vi "PH_ForceSensor.set GUI Refs.vi"(0 "VI in":refnum<vi>, 2 "GUI Refs":T1, 5 "error in (no error)":errorcluster) -> (14 "VI out":refnum<vi>, 19 "error out":errorcluster)   [LabVIEW 2014, in "PH_ForceSensor.lvlib"]
uses:
  PH_ForceSensor.lvlib
  PH_ForceSensor.GUI Refs.ctl
  PH_ForceSensor.Dataset.ctl
  PH_ForceSensor.Ranges.ctl
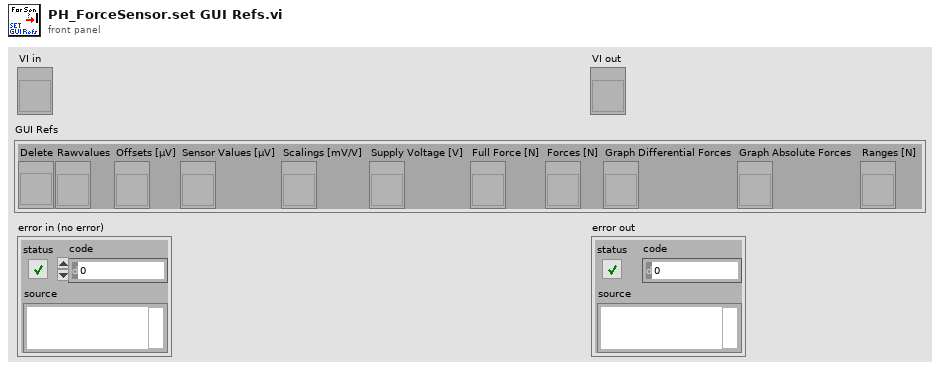
[diagram p1: front panel]
types:
  T1 = typedef "PH_ForceSensor.lvlib/PH_ForceSensor.GUI Refs.ctl" = cluster{"Delete":refnum<vi>, "Rawvalues":refnum<vi>, "Offsets [µV]":refnum<vi>, "Sensor Values [µV]":refnum<vi>, "Scalings [mV/V]":refnum<vi>, "Supply Voltage [V]":refnum<vi>, "Full Force [N]":refnum<vi>, "Forces [N]":refnum<vi>, "Graph Differential Forces":refnum<vi>, "Graph Absolute Forces":refnum<vi>, "Ranges [N]":refnum<vi>}
  T2 = typedef "PH_ForceSensor.lvlib/PH_ForceSensor.i attribute.ctl" = cluster{"GUI Refs":T1, "Rawvalues":T3, "Offsets [µV]":T3, "Scalings [mV/V]":T3, "Forces [N]":T3, "Supply Voltage [V]":dbl, "Full Force [N]":dbl, "Ranges [N]":cluster{"Low Energy":cluster{"Upper Limit":dbl, "Lower Limit":dbl}, "High Energy":cluster{"Upper Limit":dbl, "Lower Limit":dbl}}}
  T3 = typedef "PH_ForceSensor.lvlib/PH_ForceSensor.Dataset.ctl" = cluster{"top front":dbl, "top back":dbl, "bottom front":dbl, "bottom back":dbl}
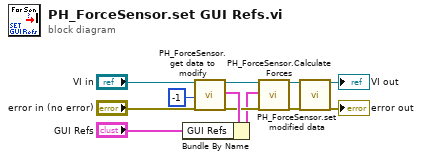
[diagram p0: block diagram]
diagram:
  n1 = call "PH_ForceSensor.get data to modify.vi"("i ref in"="VI in", "ms timeout (10000)"=-1, "error in (no error)"="error in (no error)") -> ("i ref out"=w7:refnum<vi>, "i attribute"=w12:T2, "error out"=w8:errorcluster)  [unwired: 13 in, 1 out]
  n2 = Bundle By Name(cluster=w12, "GUI Refs"="GUI Refs") -> (w6:T2)
  n3 = call "PH_ForceSensor.set modified data.vi"("i ref in"=w7, "i attribute"=w6, "error in (no error)"=w8) -> ("i ref out"=w4:refnum<vi>, "error out"=w2:errorcluster)  [unwired: 15 in]
  n4 = call "PH_ForceSensor.Calculate Forces.vi"("VI in"=w4, "error in"=w2) -> ("VI out"=→"VI out":refnum<vi>, "error out"=→"error out":errorcluster)  [unwired: 16 in]
